vi "Load Setup.vi"(8 "error in (no error)":errorcluster, 11 "JSON in":refnum<class "JSON.lvclass">) -> (0 "error out":errorcluster, 2 "Camera Setup":T1={"Exposure Time"=1e-05, "Readout Rate"=0, "Pre-amp gain"=0, "Initial Line"=1, "Final Line"=1024, "Final Column"=1024, "Initial Cloumn"=1, "Binning"=1, "EM Gain"=2, "EM Mode"=0, "Kinetic Series Length"=1} {"Kinetic Series Length" min=1; "EM Mode" items=["Electron Multiplying", "Conventional"]; "EM Gain" min=2 max=300; "Binning" min=1 max=2; "Initial Cloumn" min=1 max=1024; "Final Column" min=1 max=1024; "Final Line" min=1 max=1024; "Initial Line" min=1 max=1024; "Pre-amp gain" items=["Gain 1", "Gain 2"]; "Readout Rate" items=["30 MHz", "20 MHz", "10 MHz", "  1 MHz"]; "Exposure Time" min=1e-05}, 3 "JSON out":refnum<class "JSON.lvclass">)   [LabVIEW 2018, in "JSON.lvclass"]
uses:
  JSON.lvclass
  JSON.lvclass/JSON.ctl
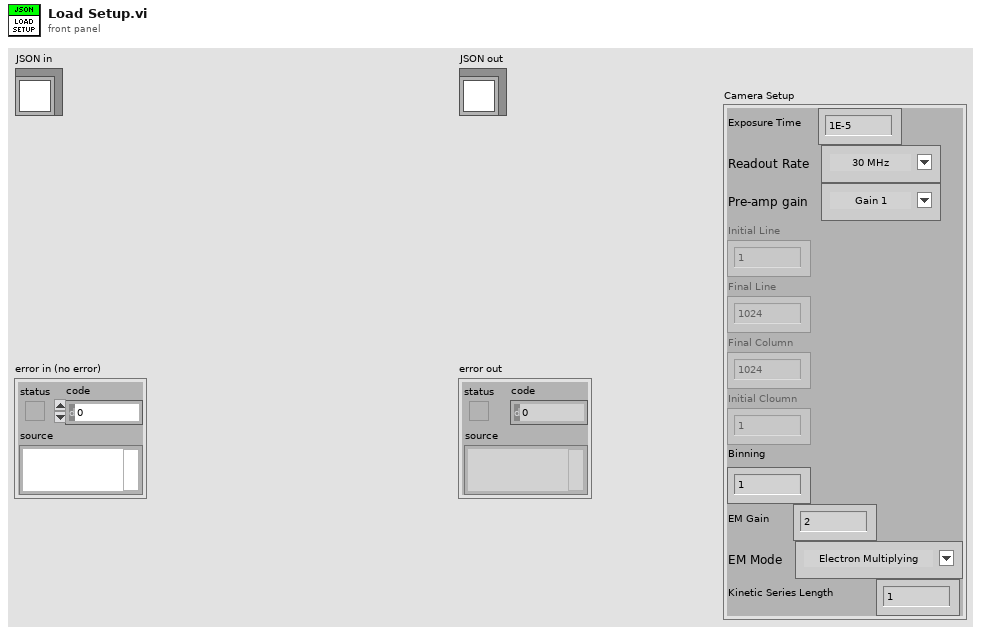
[diagram p1: front panel]
types:
  T1 = cluster{"Exposure Time":dbl, "Readout Rate":u8, "Pre-amp gain":u8, "Initial Line":u16, "Final Line":u16, "Final Column":u16, "Initial Cloumn":u16, "Binning":u8, "EM Gain":u16, "EM Mode":u8, "Kinetic Series Length":u16}
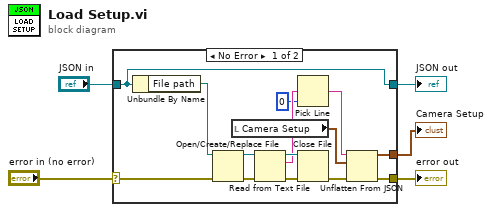
[diagram p0: block diagram]
diagram:
  n1 = case shown="No Error" "error in (no error)" {
    selector: "error in (no error)" -> [w18 w21]
    tunnel: [w11 w21] -> w4
    tunnel: [w19 w20] -> w2
    tunnel: "JSON in" -> [w19 w20]
    tunnel: [w7 _] -> w1
    frame No Error {
      n2 = Unbundle By Name(w19) -> ("File path"=w17:path)
      n3 = Open/Create/Replace File(file path (use dialog)=w17, error in=w18) -> (refnum out=w14:refnum<file>, error out=w16:errorcluster)  [unwired: 4 in, 1 out]
      n4 = local read "Camera Setup"() -> (w8:T1)
      n5 = Read from Text File(file (use dialog)=w14, error in=w16) -> (refnum out=w13:refnum<file>, text=w10:string, error out=w15:errorcluster)  [unwired: 2 in, 1 out]
      n6 = Pick Line(multi-line string=w10, line index=0) -> (output string=w9:string)  [unwired: 1 in]
      n7 = Close File(refnum=w13, error in=w15) -> (error out=w12:errorcluster)  [unwired: 1 out]
      n8 = Unflatten From JSON(JSON string=w9, type and defaults=w8, error in (no error)=w12) -> (value=w7:T1, error out=w11:errorcluster)  [unwired: 4 in]
    }
    frame Error {
    }
  }
  "error out" <- w4
  "JSON out" <- w2
  "Camera Setup" <- w1
